vi "Loop_HW.vi"() -> ()   [LabVIEW 2017, in "WCDrive2018.lvlib"]
uses:
  WCDrive2018.lvlib
  Global_SM Out Data.vi
  Global_HW_Status Out.vi
  ProtoType Code/EXAMPLE 2017 competition code/roboRIO Code/Globals/Global_HW_Address_Assignments.vi
  ENUM_ACT_State.ctl
  ENUM_ACT_Action.ctl
  _SHARE ALL/Global Share All/Global_STOP.vi
  <vilib>/Rock Robotics/WPI/MotorControl/WPI_MotorControlType.ctl
  <vilib>/Rock Robotics/SystemInterfaces/DIO/FPGA_DIOPWMChannel.ctl
  <vilib>/Rock Robotics/WPI/PWM/WPI_PWMDeadband.ctl
  <vilib>/Rock Robotics/SystemInterfaces/DIO/FPGA_DIOChannel.ctl
  <vilib>/Rock Robotics/WPI/MotorControl/WPI_MotorControlDeviceRef.ctl
  <vilib>/Rock Robotics/WPI/RobotDrive/WPI_RobotDriveDevRef.ctl
  Enum_HW Cmd Select.ctl
  Cluster_SM to HW Data.ctl
  570cffa0-ccfc-4d94-993e-2857878fdf6e.vi
panel:
  in  "SM CMD Override":bool
  in  "SM_Cmd":T1
  out "Cycle Time (S)":dbl format="%.3g"
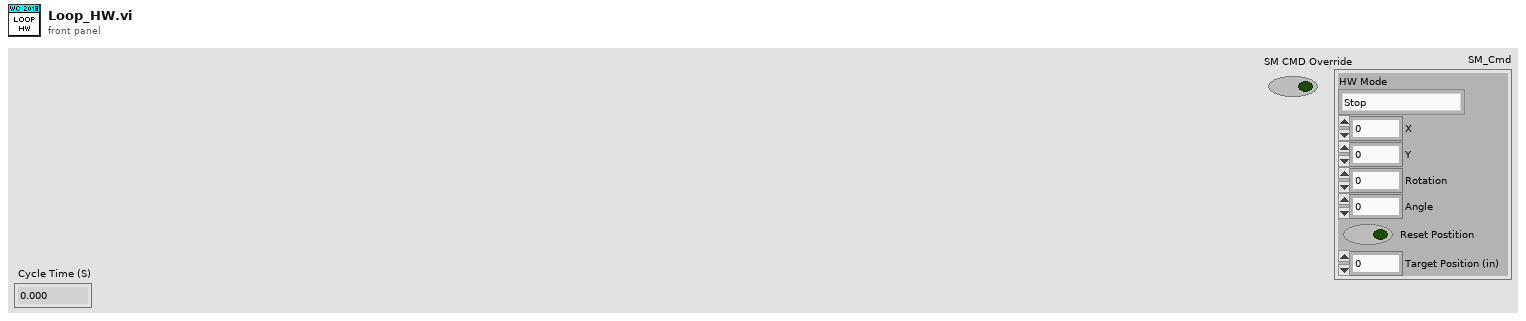
[diagram p1: front panel]
types:
  T1 = typedef "WCDrive2018.lvlib/Cluster_SM to HW Data.ctl" = cluster{"HW Mode":T2, "X":dbl, "Y":dbl, "Rotation":dbl, "Angle":dbl, "Reset Postition":bool, "Target Position (in)":dbl}
  T2 = typedef "WCDrive2018.lvlib/Enum_HW Cmd Select.ctl" = enum16{"Stop", "Vbus", "Positon Lateral", "Postition  FrontBack"}
  T3 = typedef "WPI_RobotDriveDevRef.ctl" = cluster{"DevStatus":errorcluster, "Motors[]":T4[], "Square Inputs":bool, "Max Output":dbl}
  T4 = typedef "WPI_MotorControlDeviceRef.ctl" = cluster{"DeviceStatus":errorcluster, "Type":T5, "PWM":cluster{"PWM Channel":T6, "DeadBand":T7}, "CAN":cluster{"Device Number":u8, "SetOutput VI Ref":variant, "GetOutput VI Ref":variant, "Enable VI Ref":variant, "Disable VI Ref":variant, "Data":variant}, "Invert":bool, "DIO PWM":cluster{"PWM \"Enable\" Channel":T6, "DIOChannel":T8, "PWM Rate":dbl}}
  T5 = typedef "WPI_MotorControlType.ctl" = enum16{"PWM", "CAN", "DIO PWM"}
  T6 = typedef "FPGA_DIOPWMChannel.ctl" = enum8{"PWM 0", "PWM 1", "PWM 2", "PWM 3", "PWM 4", "PWM 5", "PWM 6", "PWM 7", "PWM 8", "PWM 9", "PWM MXP 0", "PWM MXP 1", "PWM MXP 2", "PWM MXP 3", "PWM MXP 4", "PWM MXP 5", "PWM MXP 6", "PWM MXP 7", "PWM MXP 8", "PWM MXP 9", "Invalid"}
  T7 = typedef "WPI_PWMDeadband.ctl" = cluster{"Name":string, "maxPositivePwm":i32, "minPositivePwm":i32, "centerPwm":i32, "maxNegativePwm":i32, "minNegativePwm":i32, "angularRange":u16}
  T8 = typedef "FPGA_DIOChannel.ctl" = enum8{"DIO 0", "DIO 1", "DIO 2", "DIO 3", "DIO 4", "DIO 5", "DIO 6", "DIO 7", "DIO 8", "DIO 9", "DIO MXP 0", "DIO MXP 1", "DIO MXP 2", "DIO MXP 3", "DIO MXP 4", "DIO MXP 5", "DIO MXP 6", "DIO MXP 7", "DIO MXP 8", "DIO MXP 9", "DIO MXP 10", "DIO MXP 11", "DIO MXP 12", "DIO MXP 13", "DIO MXP 14", "DIO MXP 15", "SPI Port CS1", "SPI Port CS2", "SPI Port CS3", "SPI Port MISO", "SPI Port MOSI", "Invalid"}
  T9 = typedef "WCDrive2018.lvlib/ENUM_ACT_State.ctl" = enum16{"_Startup", "_Idle", "_Shutdown"}
  T10 = typedef "WCDrive2018.lvlib/ENUM_ACT_Action.ctl" = enum16{"No Action", "Reset Time", "Reset All", "Initialize SRXs", "_Action B"}
  T11 = typedef "Cluster_WCDrive_SetupData.ctl" = cluster{"Left Master":u8, "Invert Left Master":bool, "Left Slave":u8, "Invert Left Slave":bool, "Right Master":u8, "Invert Right Master":bool, "Right Slave":u8, "Invert Right Slave":bool, "Invert Left Encoder":bool, "Invert Right Encoder":bool}
  T12 = cluster{"State":T9, "Previous State":T9, "Current Time":timestamp, "Previous Time":timestamp, "Start Time":timestamp, "Target Time (ms)":u32, "Cycle Time(S)":dbl, "RobotDriveDevRef":T3, "SM_Cmd":T1, "HW SETUP_WC Drive":T11}
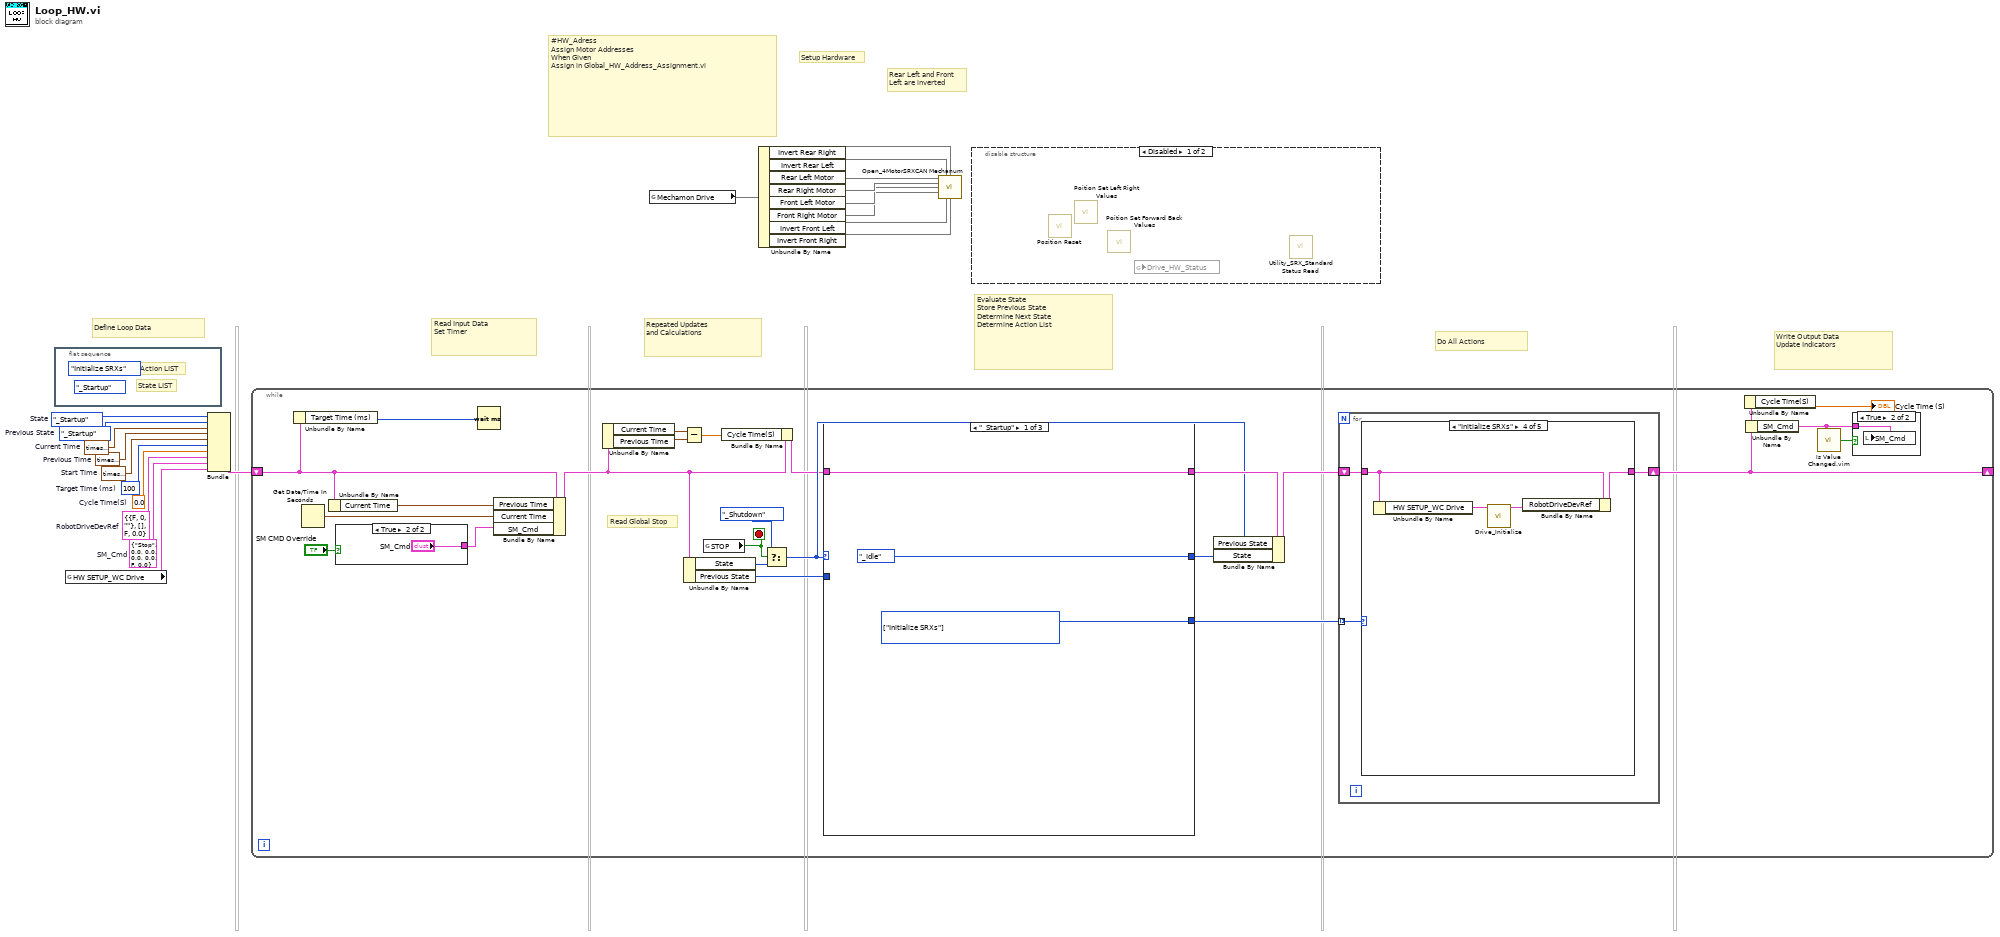
[diagram p0: block diagram]
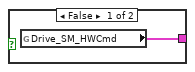
[diagram p2: hidden frame]
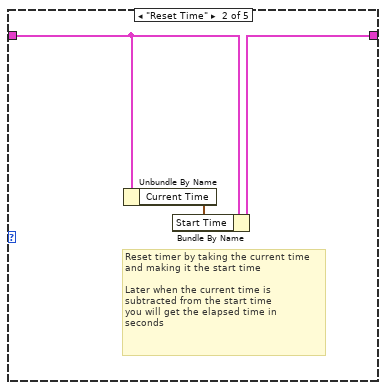
[diagram p5: hidden frame]
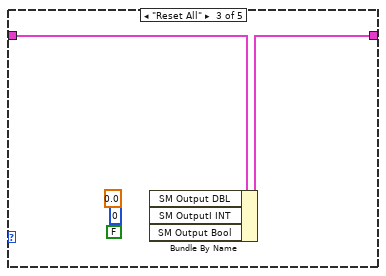
[diagram p6: hidden frame]
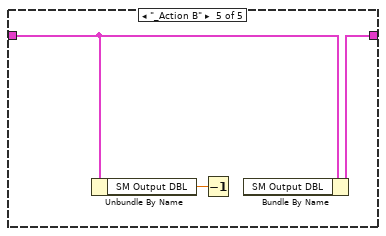
[diagram p7: hidden frame]
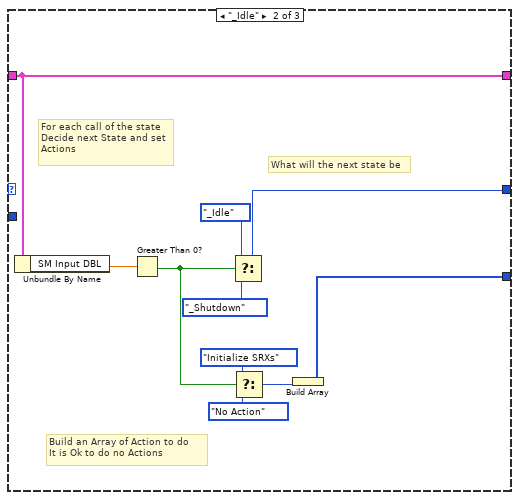
[diagram p8: hidden frame]
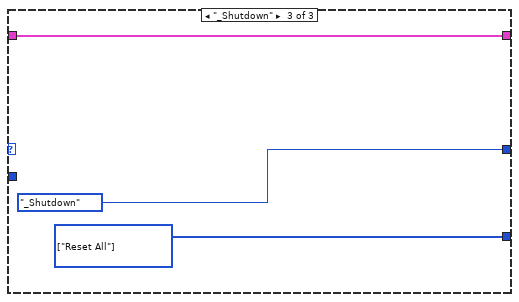
[diagram p9: hidden frame]
diagram:
  w2 = T1 {"HW Mode"=enum."Stop", "X"=0.0, "Y"=0.0, "Rotation"=0.0, "Angle"=0.0, "Reset Postition"=FALSE, "Target Position (in)"=0.0}  # SM_Cmd
  w3 = T3 {"DevStatus"={"status"=FALSE, "code"=0, "source"=""}, "Motors[]"=[], "Square Inputs"=FALSE, "Max Output"=0.0}  # RobotDriveDevRef
  w4 = 0.0  # Cycle Time(S)
  w5 = ENUM_ACT_State."_Startup"  # Previous State
  w6 = timestamp(0 s since 1904-01-01)  # Previous Time
  w7 = u32 100  # Target Time (ms)
  w8 = timestamp(0 s since 1904-01-01)  # Start Time
  w9 = timestamp(0 s since 1904-01-01)  # Current Time
  w10 = ENUM_ACT_State."_Startup"  # State
  # "Define Loop Data"
  # "Repeated Updates\nand Calculations"
  # "Read Input Data\nSet Timer"
  # "Evaluate State\nStore Previous State\nDetermine Next State\nDetermine Action List"
  # "Do All Actions"
  # "Write Output Data\nUpdate Indicators"
  # "#HW_Adress\nAssign Motor Addresses\nWhen Given\nAssign in Global_HW_Address_Assignment.vi"
  # "Rear Left and Front \nLeft are inverted"
  # "Setup Hardware"
  n1 = flat-sequence {
    frame #0 {
      (unwired) ENUM_ACT_State."_Startup" ("State")
      (unwired) ENUM_ACT_Action."Initialize SRXs" ("Action")
      # "State LIST"
      # "Action LIST"
    }
  }
  n2 = global read "Global_HW_Address_Assignments.vi" "HW SETUP_WC Drive"() -> (w1:T11)
  n3 = Bundle("State"=w10, "Previous State"=w5, "Current Time"=w9, "Previous Time"=w6, "Start Time"=w8, "Target Time (ms)"=w7, "Cycle Time(S)"=w4, "RobotDriveDevRef"=w3, "SM_Cmd"=w2, "HW SETUP_WC Drive"=w1) -> (w11:T12)  [unwired: 1 in]
  n4 = while {
    shift-right: [w32] -> _
    shift-left: w11 -> [w35]
    stop <- w40 stop-if-true
    # "Read Global Stop"
    n5 = Unbundle By Name(w35) -> ("Target Time (ms)"=w37:u32)
    n6 = Get Date/Time In Seconds() -> (seconds since 1Jan1904=w44:timestamp)
    n7 = Unbundle By Name(w35) -> ("Current Time"=w36:timestamp)
    n8 = case shown="True" "SM CMD Override" {
      tunnel: [w45 "SM_Cmd"] -> w24
      frame False {
        n9 = global read "Global_SM Out Data.vi" "Drive_SM_HWCmd"() -> (w45:T1)
      }
      frame True {
      }
    }
    n10 = Wait (ms)(milliseconds to wait=w37) -> ()  [unwired: 1 out]
    n11 = Bundle By Name(cluster=w35, "Previous Time"=w36, "Current Time"=w44, "SM_Cmd"=w24) -> (w28:T12)
    n12 = Unbundle By Name(w28) -> ("Current Time"=w29:timestamp, "Previous Time"=w30:timestamp)
    n13 = Subtract(x=w29, y=w30) -> (x-y=w26:dbl)
    n14 = Unbundle By Name(w28) -> ("State"=w38:T9, "Previous State"=w34:T9)
    n15 = global read "Global_STOP.vi" "STOP"() -> (w40:bool)
    n16 = Bundle By Name(cluster=w28, "Cycle Time(S)"=w26) -> (w27:T12)
    n17 = Select(t=ENUM_ACT_State."_Shutdown" ("State"), s=w40, f=w38) -> (s? t:f=w33:T9)
    n18 = case shown="\"_Startup\"" w33 {
      tunnel: w27 -> [w66 w76 w79]
      tunnel: [w66 w76 w79] -> w42
      tunnel: [ENUM_ACT_State."_Idle" ("State") w74 ENUM_ACT_State."_Shutdown" ("State")] -> w41
      tunnel: [w65 w67 w77] -> w25
      tunnel: w34 -> [_ _ _]
      frame "_Startup" {
        w65 = T10[] [enum."Initialize SRXs"] items=["No Action", "Reset Time", "Reset All", "Initialize SRXs", "_Action B"] ("Actions")
      }
      frame "_Idle" {
        # "For each call of the state\nDecide next State and set\nActions"
        # "What will the next state be"
        # "Build an Array of Action to do\nIt is Ok to do no Actions"
        n19 = Unbundle By Name(w76) -> ("SM Input DBL"=w75:dbl)
        n20 = Greater Than 0?(x=w75) -> (x > 0?=w69:bool)
        n21 = Select(t=ENUM_ACT_State."_Idle" ("State"), s=w69, f=ENUM_ACT_State."_Shutdown" ("State")) -> (s? t:f=w74:T9)
        n22 = Select(t=ENUM_ACT_Action."Initialize SRXs" ("Action"), s=w69, f=ENUM_ACT_Action."No Action" ("Action")) -> (s? t:f=w68:T10)
        n23 = Build Array(w68) -> (w67:T10[])
      }
      frame "_Shutdown" {
        w77 = T10[] [enum."Reset All"] items=["No Action", "Reset Time", "Reset All", "Initialize SRXs", "_Action B"] ("Actions")
      }
    }
    n24 = Bundle By Name(cluster=w42, "Previous State"=w33, "State"=w41) -> (w43:T12)
    n25 = for {
      tunnel: w25 -> [w50] mode=indexing
      shift-right: [w49] -> w32
      shift-left: w43 -> [w48]
      n26 = case shown="\"Initialize SRXs\"" w50 {
        tunnel: w48 -> [w51 w54 w56 w58 w62]
        tunnel: [w51 w53 w55 w59 w61] -> w49
        frame "No Action" {
        }
        frame "Reset Time" {
          # "Reset timer by taking the current time\nand making it the start time\n\nLater when the current time is \nsubtracted from the start time\nyou will get the elapsed time in \nseconds"
          n27 = Unbundle By Name(w54) -> ("Current Time"=w52:timestamp)
          n28 = Bundle By Name(cluster=w54, "Start Time"=w52) -> (w53:T12)
        }
        frame "Reset All" {
          (unwired) FALSE ("Output Bool")
          (unwired) 0 ("OutputI INT")
          (unwired) 0.0 ("FG Write Value")
          n29 = Bundle By Name(cluster=w56) -> (w55:T12)  [unwired: 3 in]
        }
        frame "Initialize SRXs" {
          n30 = Unbundle By Name(w58) -> ("HW SETUP_WC Drive"=w57:T11)
          n31 = call "Drive_Initialize.vi"("HW SETUP_WC Drive"=w57) -> ("RobotDriveDevRef Out"=w60:T3)  [unwired: 10 in]
          n32 = Bundle By Name(cluster=w58, "RobotDriveDevRef"=w60) -> (w59:T12)
        }
        frame "_Action B" {
          n33 = Unbundle By Name(w62) -> ("SM Output DBL"=w63:dbl)
          n34 = Decrement(x=w63) -> ()  [unwired: 1 out]
          n35 = Bundle By Name(cluster=w62) -> (w61:T12)  [unwired: 1 in]
        }
      }
    }
    n36 = Unbundle By Name(w32) -> ("Cycle Time(S)"=→"Cycle Time (S)":dbl)
    n37 = Unbundle By Name(w32) -> ("SM_Cmd"=w22:T1)
    n38 = call "Is Value Changed.vim"("value"=w22) -> ("changed or first call?"=w23:bool)
    n39 = case shown="True" w23 {
      tunnel: w22 -> [_ w47]
      frame False {
      }
      frame True {
        n40 = local write "SM_Cmd"(w47) -> ()
      }
    }
  }
  n41 = global read "Global_HW_Address_Assignments.vi" "Mechamon Drive"() -> (w20)
  n42 = Unbundle By Name(w20) -> ("Invert Rear Right"=w19, "Invert Rear Left"=w18, "Rear Left Motor"=w17, "Rear Right Motor"=w14, "Front Left Motor"=w13, "Front Right Motor"=w12, "Invert Front Left"=w15, "Invert Front Right"=w16)
  n43 = call "Open_4MotorSRXCAN Mechanum.vi"("Rear Left Motor"=w17, "Rear Left Motor Inverted"=w18, "Rear Right Motor Inverted"=w19, "Rear Right Motor"=w14, "Front Left Motor"=w13, "Front Right Motor"=w12, "Front Left Motor Inverted"=w15, "Front Right Motor Inverted"=w16) -> ()  [unwired: 6 in, 2 out]
  n44 = disable-structure shown="Disabled" {
    frame Disabled {
      n45 = call "Position Reset.vi"() -> ()  [unwired: 10 in, 2 out]
      n46 = call "Poition Set Left Right Values.vi"() -> ()  [unwired: 10 in, 2 out]
      n47 = call "Poition Set Forward Back Values.vi"() -> ()  [unwired: 10 in, 2 out]
      n48 = global read "Global_HW_Status Out.vi" "Drive_HW_Status"() -> ()  [unwired: 1 in]
      n49 = call "Utility_SRX_Standard Status Read.vi"() -> ()  [unwired: 9 in, 3 out]
    }
    frame Enabled {
    }
  }
